vi "Strings Global.vi"() -> ()   [LabVIEW 2015, in "NI_Azure_Blob.lvlib"]
uses:
  NI_Azure_Blob.lvlib
panel:
  in  "Warning.BreakDuration":string="Requested break duration was out of range and coerced to a valid range of 0 to 60 seconds."
  in  "Warning.LeaseDuration":string="Requested lease duration was out of range and coerced to a valid range of 15 to 60 seconds."
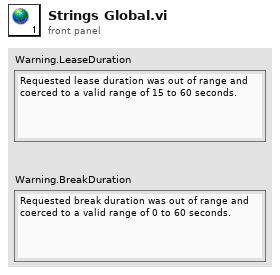
[diagram p1: front panel]
diagram:
